vi "Ltree to JSON.vi"(10 "Values":string[](array[string]), 11 "Names":string[](array[string])) -> (3 "JSON String":string)   [LabVIEW 2019, in "Userlib.lvlib"]
uses:
  Userlib.lvlib
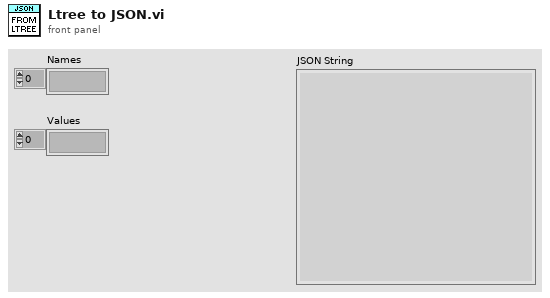
[diagram p1: front panel]
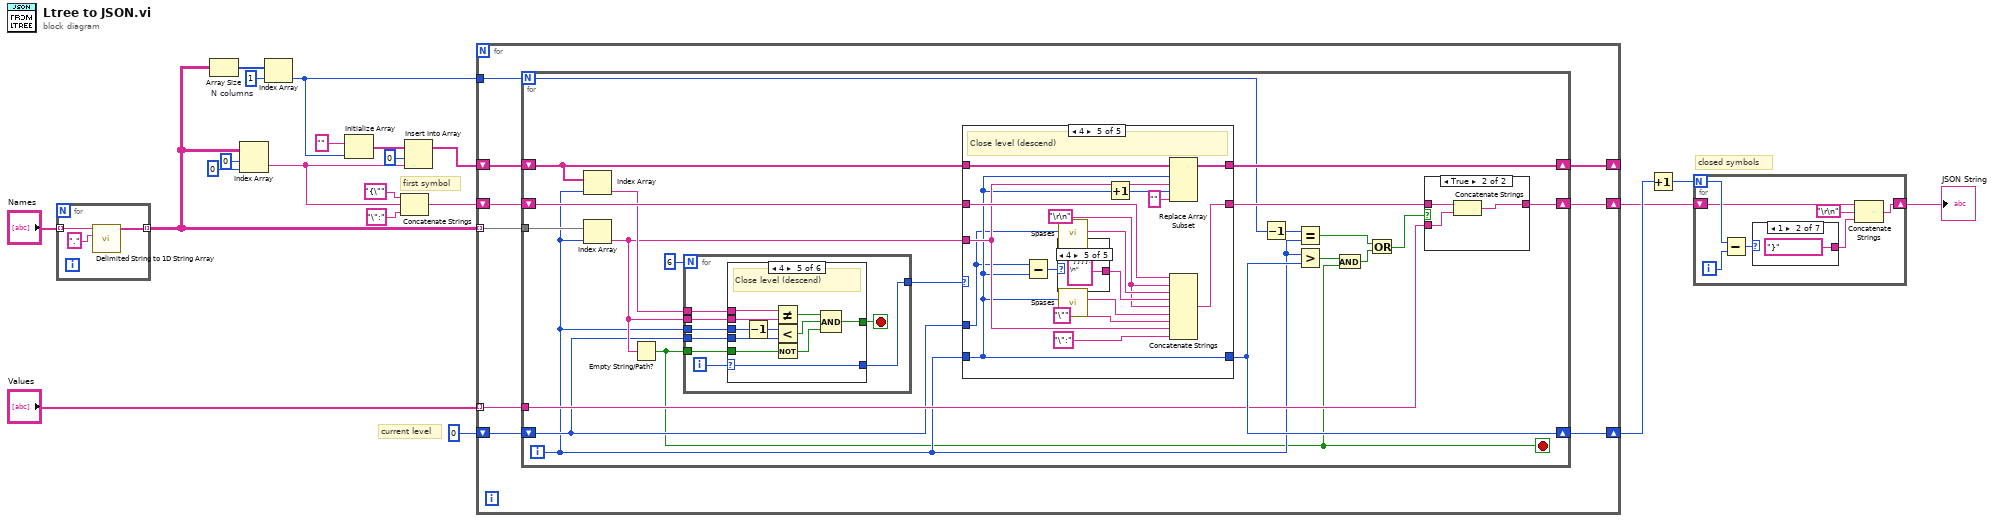
[diagram p0: block diagram]
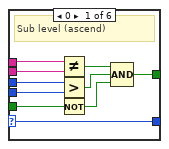
[diagram p2: hidden frame]
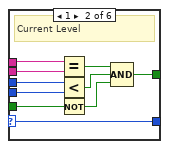
[diagram p3: hidden frame]
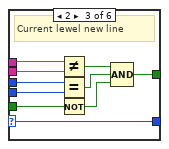
[diagram p4: hidden frame]
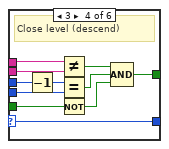
[diagram p5: hidden frame]
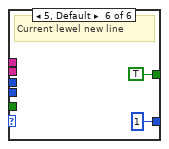
[diagram p6: hidden frame]
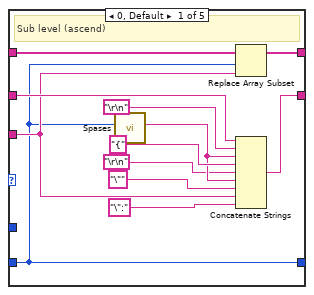
[diagram p7: hidden frame]
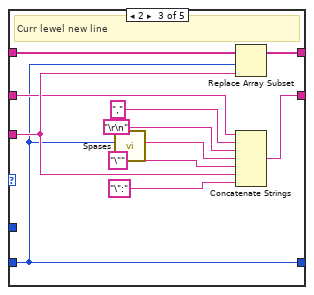
[diagram p9: hidden frame]
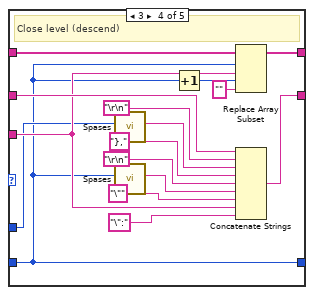
[diagram p10: hidden frame]
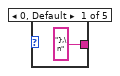
[diagram p11: hidden frame]
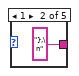
[diagram p12: hidden frame]
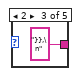
[diagram p13: hidden frame]
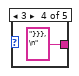
[diagram p14: hidden frame]
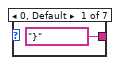
[diagram p16: hidden frame]
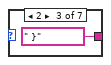
[diagram p17: hidden frame]
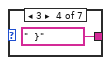
[diagram p18: hidden frame]
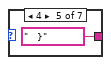
[diagram p19: hidden frame]
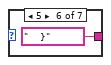
[diagram p20: hidden frame]
diagram:
  w19 = 1  # N columns
  # "closed symbols"
  # "first symbol"
  # "current level"
  n1 = for {
    tunnel: [w22] -> w1 mode=indexing
    tunnel: "Names" -> [w23] mode=indexing
    n2 = call <vilib>:"Delimited String to 1D String Array.vi"("delimiter"="." ("delimiter (Tab)"), "delimited string"=w23) -> ("string array"=w22:string[])  [unwired: 9 in]
  }
  n3 = Array Size(array=w1) -> (size(s)=w20:i32[])
  n4 = Index Array(array=w1, index (row)=0, index (col)=0 ("disabled index (col)")) -> (element=w12:string)
  n5 = Index Array(array=w20, index=w19) -> (element=w7:i32)
  n6 = Initialize Array("", w7) -> (w14:string[])
  n7 = Concatenate Strings("{\"", w12, "\":" ("string")) -> (w15:string)
  n8 = Insert Into Array(array=w14, index=0, new element=w12) -> (w11:string[])
  n9 = for {
    tunnel: w1 -> [w30] mode=indexing
    shift-right: [w31] -> w9
    shift-left: w15 -> [w32]
    shift-right: [w28] -> w10
    shift-left: 0 -> [w29]
    shift-right: [w27] -> _
    shift-left: w11 -> [w33]
    tunnel: w7 -> [w26]
    tunnel: "Values" -> [w25] mode=indexing
    n10 = for {
      N: w26 -> [w38]
      tunnel: w30 -> [w51]
      shift-right: [w53] -> w27
      shift-left: w33 -> [w54]
      shift-right: [w49] -> w31
      shift-left: w32 -> [w52]
      shift-right: [w47] -> w28
      shift-left: w29 -> [w43]
      tunnel: w25 -> [w46]
      i -> [w39]
      stop <- w34 stop-if-true
      n11 = Index Array(array=w54, index=w39) -> (element=w45:string)
      n12 = Index Array(array=w51, index=w39) -> (element=w44:string)
      n13 = Empty String/Path?(string/path=w44) -> (empty?=w34:bool)
      n14 = for {
        N: 6 -> [_]
        tunnel: w45 -> [w62]
        tunnel: w44 -> [w61]
        tunnel: w43 -> [w60]
        tunnel: w34 -> [w59]
        tunnel: w39 -> [w58]
        tunnel: [w55] -> w42
        i -> [w56]
        stop <- w57 stop-if-true
        n15 = case shown="4" w56 {
          selector: w56 -> [w63 w73 w83 w93 w104 _]
          tunnel: w62 -> [w69 w79 w89 w100 w111 _]
          tunnel: w61 -> [w68 w78 w88 w99 w110 _]
          tunnel: w58 -> [w67 w77 w87 w95 w106 _]
          tunnel: w60 -> [w66 w76 w86 w98 w109 _]
          tunnel: w59 -> [w65 w75 w85 w97 w108 _]
          tunnel: [w64 w74 w84 w96 w107 TRUE] -> w57
          tunnel: [w63 w73 w83 w93 w104 1] -> w55
          frame 0 {
            # "Sub level (ascend)"
            n16 = Not Equal?(x=w69, y=w68) -> (x != y?=w72:bool)
            n17 = Greater?(x=w67, y=w66) -> (0:w71:bool)
            n18 = Not(x=w65) -> (.not. x?=w70:bool)
            n19 = Compound Arithmetic op=AND(w72, w71, w70) -> (w64:bool)
          }
          frame 1 {
            # "Current Level"
            n20 = Equal?(x=w79, y=w78) -> (x = y?=w82:bool)
            n21 = Less?(x=w77, y=w76) -> (x < y?=w81:bool)
            n22 = Not(x=w75) -> (.not. x?=w80:bool)
            n23 = Compound Arithmetic op=AND(w82, w81, w80) -> (w74:bool)
          }
          frame 2 {
            # "Current lewel new line"
            n24 = Not Equal?(x=w89, y=w88) -> (x != y?=w92:bool)
            n25 = Equal?(x=w87, y=w86) -> (x = y?=w91:bool)
            n26 = Not(x=w85) -> (.not. x?=w90:bool)
            n27 = Compound Arithmetic op=AND(w92, w91, w90) -> (w84:bool)
          }
          frame 3 {
            # "Close level (descend)"
            n28 = Decrement(x=w95) -> (x-1=w94:i32)
            n29 = Not Equal?(x=w100, y=w99) -> (x != y?=w103:bool)
            n30 = Equal?(x=w94, y=w98) -> (x = y?=w102:bool)
            n31 = Not(x=w97) -> (.not. x?=w101:bool)
            n32 = Compound Arithmetic op=AND(w103, w102, w101) -> (w96:bool)
          }
          frame 4 {
            # "Close level (descend)"
            n33 = Decrement(x=w106) -> (x-1=w105:i32)
            n34 = Not Equal?(x=w111, y=w110) -> (x != y?=w114:bool)
            n35 = Less?(x=w105, y=w109) -> (x < y?=w113:bool)
            n36 = Not(x=w108) -> (.not. x?=w112:bool)
            n37 = Compound Arithmetic op=AND(w114, w113, w112) -> (w107:bool)
          }
          frame 5, Default {
            # "Current lewel new line"
          }
        }
      }
      n38 = case shown="4" w42 {
        tunnel: w44 -> [w123 _ w138 w152 w169]
        tunnel: [w128 w131 w142 w158 w174] -> w50
        tunnel: w54 -> [w127 w129 w141 w157 w173]
        tunnel: w39 -> [w119 _ w133 w145 w163]
        tunnel: [w126 w129 w140 w156 w172] -> w53
        tunnel: w52 -> [w125 w131 w135 w155 w171]
        tunnel: w43 -> [_ w130 _ w147 w162]
        tunnel: [w119 w130 w133 w145 w163] -> w47
        frame 0, Default {
          # "Sub level (ascend)"
          n39 = call "Spases.vi"("Numeric"=w119) -> ("spaces"=w118:string)  [unwired: 10 in]
          n40 = Replace Array Subset(array=w127, new element=w123, index=w119) -> (w126:string[])
          n41 = Concatenate Strings(w125, "\r\n", w118, "{", "\r\n", w118, "\"", w123, "\":" ("string")) -> (w128:string)
        }
        frame 1 {
          # "Current Level"
        }
        frame 2 {
          # "Curr lewel new line"
          n42 = call "Spases.vi"("Numeric"=w133) -> ("spaces"=w132:string)  [unwired: 10 in]
          n43 = Replace Array Subset(array=w141, new element=w138, index=w133) -> (w140:string[])
          n44 = Concatenate Strings(w135, ",", "\r\n", w132, "\"", w138, "\":" ("string")) -> (w142:string)
        }
        frame 3 {
          # "Close level (descend)"
          n45 = call "Spases.vi"("Numeric"=w147) -> ("spaces"=w146:string)  [unwired: 10 in]
          n46 = call "Spases.vi"("Numeric"=w145) -> ("spaces"=w144:string)  [unwired: 10 in]
          n47 = Increment(x=w145) -> (x+1=w149:i32)
          n48 = Replace Array Subset(array=w157, new element #1=w152, index #1=w145, new element #2="" ("new element/subarray"), index #2=w149) -> (w156:string[])
          n49 = Concatenate Strings(w155, "\r\n", w146, "},", "\r\n", w144, "\"", w152, "\":" ("string")) -> (w158:string)
        }
        frame 4 {
          w159 = "\r\n"
          # "Close level (descend)"
          n50 = Subtract(x=w162, y=w163) -> (x-y=w167:i32)
          n51 = case shown="4" w167 {
            tunnel: ["},\n" "},\n" "}},\n" "}}},\n" "}}}},\n"] -> w166
            frame 0, Default {
            }
            frame 1 {
            }
            frame 2 {
            }
            frame 3 {
            }
            frame 4 {
            }
          }
          n52 = call "Spases.vi"("Numeric"=w162) -> ("spaces"=w161:string)  [unwired: 10 in]
          n53 = call "Spases.vi"("Numeric"=w163) -> ("spaces"=w160:string)  [unwired: 10 in]
          n54 = Increment(x=w163) -> (x+1=w165:i32)
          n55 = Replace Array Subset(array=w173, new element #1=w169, index #1=w163, new element #2="" ("new element/subarray"), index #2=w165) -> (w172:string[])
          n56 = Concatenate Strings(w171, w159, w161, w166, w159, w160, "\"", w169, "\":" ("string")) -> (w174:string)
        }
      }
      n57 = Decrement(x=w38) -> (x-1=w40:i32)
      n58 = Equal?(x=w40, y=w39) -> (x = y?=w36:bool)
      n59 = Greater?(x=w39, y=w47) -> (0:w35:bool)
      n60 = And(x=w35, y=w34) -> (x .and. y?=w48:bool)
      n61 = Or(x=w36, y=w48) -> (x .or. y?=w37:bool)
      n62 = case shown="True" w37 {
        tunnel: w50 -> [w180 w183]
        tunnel: [w180 w181] -> w49
        tunnel: w46 -> [_ w182]
        frame False {
        }
        frame True {
          n63 = Concatenate Strings(w183, w182) -> (w181:string)
        }
      }
    }
  }
  n64 = Increment(x=w10) -> (x+1=w6:i32)
  n65 = for {
    N: w6 -> [w190]
    shift-right: [w186] -> w3
    shift-left: w9 -> [w187]
    i -> [w189]
    n66 = Subtract(x=w190, y=w189) -> (x-y=w188:i32)
    n67 = case shown="1" w188 {
      tunnel: ["}" ("end") "}" ("end") " }" ("end") "  }" ("end") "   }" ("end") "    }" ("end") "     }" ("end")] -> w184
      frame 0, Default {
      }
      frame 1 {
      }
      frame 2 {
      }
      frame 3 {
      }
      frame 4 {
      }
      frame 5 {
      }
      frame 6 {
      }
    }
    n68 = Concatenate Strings(w187, "\r\n", w184) -> (w186:string)
  }
  "JSON String" <- w3
